vi "Get Port Frames.vi"(8 "error in":errorcluster, 11 "Port Ref":T1 format="%.0x") -> (0 "error out":errorcluster, 1 "Outgoing Frames":T1[](array[typedef]) format="%.0x", 2 "Incoming Frames":T1[](array[typedef]) format="%.0x", 3 "Port Ref out":T1 format="%.0x")   [LabVIEW 2020, in "Communication Bus Template Scripting.lvlib"]
uses:
  <vilib>/NI VeriStand/Custom Device API/Custom Device Item Ref.ctl
  Communication Bus Template Scripting.lvlib
  <vilib>/NI VeriStand/Custom Device Tools/Custom Device Utility Library/Custom Device Utility Library.lvlib
  <vilib>/NI VeriStand/Custom Device Tools/Custom Device Utility Library/NI VeriStand - Search for All Items by GUID.vi
  Constants.vi
  <vilib>/NI VeriStand/Custom Device API/Custom Device API.lvlib
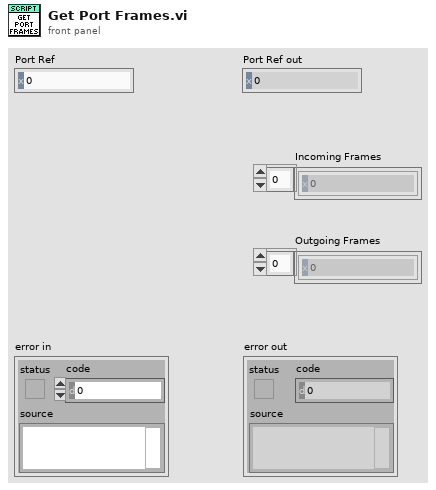
[diagram p1: front panel]
types:
  T1 = typedef "Custom Device API.lvlib/Custom Device Item Ref.ctl" = u64
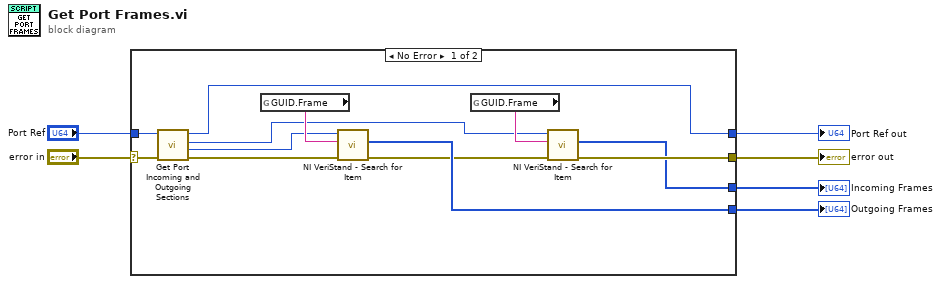
[diagram p0: block diagram]
diagram:
  n1 = case shown="No Error" "error in" {
    selector: "error in" -> [w17 w20]
    tunnel: "Port Ref" -> [w18 w19]
    tunnel: [w8 w20] -> w5
    tunnel: [w11 w19] -> w4
    tunnel: [w7 _] -> w1
    tunnel: [w14 _] -> w2
    frame No Error {
      n2 = call "Get Port Incoming and Outgoing Sections.vi"("error in"=w17, "Port Ref"=w18) -> ("error out"=w15:errorcluster, "Outgoing"=w9:T1, "Incoming"=w10:T1, "Port Ref out"=w11:T1)  [unwired: 6 in]
      n3 = global read "Constants.vi" "GUID.Frame"() -> (w16:string)
      n4 = call-poly <vilib>:"NI VeriStand - Search for Item.vi"("error in"=w15, "Item GUID"=w16, "Section Ref in"=w9) -> ("error out"=w12:errorcluster, "Item Refs"=w14:T1[])  [unwired: 5 in, 2 out]
      n5 = global read "Constants.vi" "GUID.Frame"() -> (w13:string)
      n6 = call-poly <vilib>:"NI VeriStand - Search for Item.vi"("error in"=w12, "Item GUID"=w13, "Section Ref in"=w10) -> ("error out"=w8:errorcluster, "Item Refs"=w7:T1[])  [unwired: 5 in, 2 out]
    }
    frame Error {
    }
  }
  "error out" <- w5
  "Port Ref out" <- w4
  "Incoming Frames" <- w1
  "Outgoing Frames" <- w2
